vi "IMU Get Yaw Wrapper.vi"   [LabVIEW 2026, in "MrcLib.lvlib"]
uses:
  MrcLib.lvlib
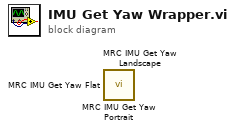
[diagram p0: block diagram]
diagram:
  n1 = call <vilib>:"MRC IMU Get Yaw Portrait.vi"() -> ()  [unwired: 8 in, 4 out]
  n2 = call <vilib>:"MRC IMU Get Yaw Landscape.vi"() -> ()  [unwired: 8 in, 4 out]
  n3 = call "MRC IMU Get Yaw Flat.vi"() -> ()  [unwired: 9 in, 3 out]
